vi "Sample Client.vi"() -> ()   [LabVIEW 2021]
uses:
  CIF_PluginLoader_client/RPC Messages/cif_manager_LoaderStatus.ctl
  CIF_PluginLoader_client/RPC Messages/cif_manager_LoaderInfo.ctl
  CIF_PluginLoader_client/RPC Messages/cif_manager_LoaderType.ctl
  CIF_Plugin_Loader_Client_Wrapper/CIFPluginLoaderClientWrapper.lvlib
  CIF_PluginLoader_client/CIF_PluginLoader_client.lvlib
panel:
  out "Loader Status":T1
  out "error out":errorcluster
  in  "address":string="localhost:"
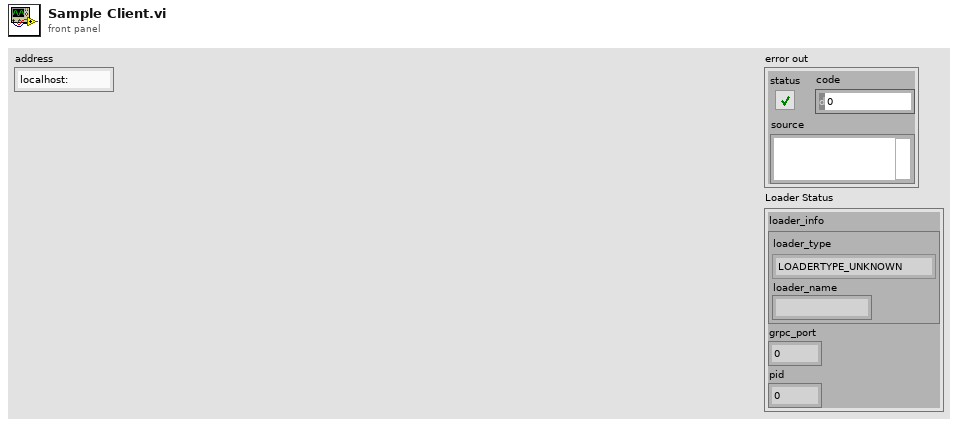
[diagram p1: front panel]
types:
  T1 = typedef "CIF_PluginLoader_client.lvlib/cif_manager_LoaderStatus.ctl" = cluster{"loader_info":T2, "grpc_port":i32, "pid":u32}
  T2 = typedef "CIF_PluginLoader_client.lvlib/cif_manager_LoaderInfo.ctl" = cluster{"loader_type":T3, "loader_name":string}
  T3 = typedef "CIF_PluginLoader_client.lvlib/cif_manager_LoaderType.ctl" = enum32{"LOADERTYPE_UNKNOWN", "LOADERTYPE_LABVIEW"}
  T4 = typedef "grpc-lvsupport-release.lvlib/grpcId.ctl" = u64
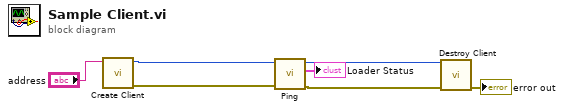
[diagram p0: block diagram]
diagram:
  n1 = call "Create Client.vi"("address"="address") -> ("error out"=w4:errorcluster, "gRPC ID Out"=w5:T4)  [unwired: 9 in]
  n2 = call "Ping.vi"("error in"=w4, "gRPC ID in"=w5) -> ("error out"=w6:errorcluster, "Loader Status"=→"Loader Status":T1, "gRPC ID out"=w7:T4)  [unwired: 7 in]
  n3 = call "Destroy Client.vi"("error in"=w6, "gRPC ID"=w7) -> ("error out"=→"error out":errorcluster)  [unwired: 9 in]
